vi "Constants.vi"() -> ()   [LabVIEW 2021, in "Large Number Operation Shared.lvlib"]
doc: "Use this Global VI to access the GUIDs assigned to the page resources of the Custom Device."
uses:
  Large Number Operation Shared.lvlib
panel:
  in  "Tab Control":enum32{"GUIDs", "Constants", "Properties"}(tab)
  in  "Large Number Operation":string="03d356e4-9bf2-43b5-af92-00f39b761305"
  in  "Compiled.Settings":string="Compiled.Settings"
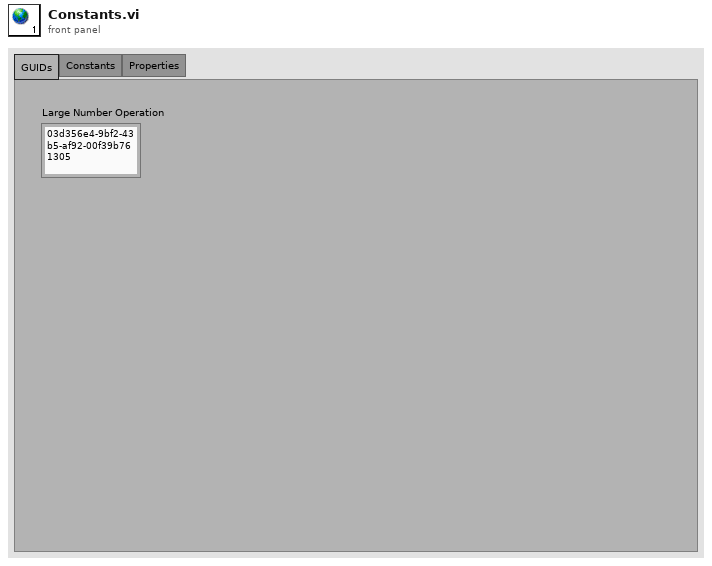
[diagram p1: front panel]
diagram:
